vi "Route Specification to Connected Routes Listbox.vi"(8 "error in (no error)":errorcluster, 10 "route specification":string, 11 "listbox reference":refnum<vi>) -> (0 "error out":errorcluster, 3 "listbox reference out":refnum<vi>)   [LabVIEW 2023, in "SwitchExecController.lvlib"]
uses:
  SwitchExecController.lvlib
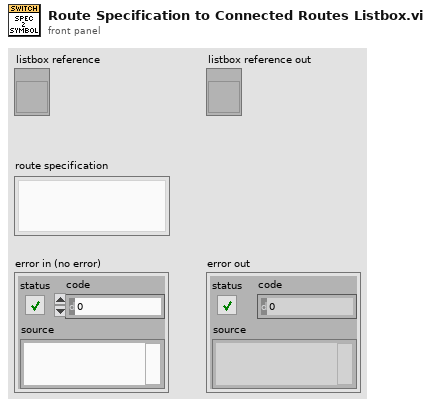
[diagram p1: front panel]
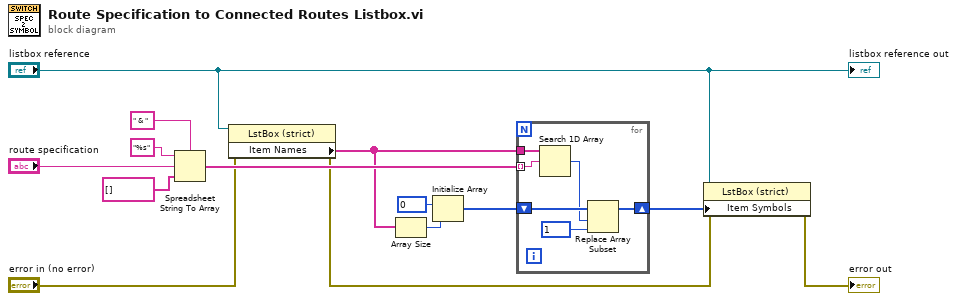
[diagram p0: block diagram]
diagram:
  n1 = Spreadsheet String To Array(delimiter (Tab)=" & ", format string="%s", spreadsheet string="route specification", array type (2D Dbl)=string[] []) -> (array=w10:string[])
  n2 = property class="LstBox (strict)"(reference="listbox reference", error in="error in (no error)") -> (error out=w3:errorcluster, "Item Names"=w7:string[])  [unwired: 1 out]
  n3 = Array Size(array=w7) -> (size(s)=w9:i32)
  n4 = Initialize Array(0, w9) -> (w6:i32[])
  n5 = for {
    tunnel: w10 -> [w19] mode=indexing
    tunnel: w7 -> [w20]
    shift-right: [w15] -> w5
    shift-left: w6 -> [w18]
    n6 = Search 1D Array(1D array=w20, element=w19) -> (index of element=w17:i32)  [unwired: 1 in]
    n7 = Replace Array Subset(array=w18, new element=1, index=w17) -> (w15:i32[])
  }
  n8 = property class="LstBox (strict)"(reference="listbox reference", error in=w3, "Item Symbols"=w5) -> (error out=→"error out":errorcluster)  [unwired: 1 out]
  "listbox reference out" <- "listbox reference"
